vi "Chamber controller RT SAVE.vi"() -> ()   [LabVIEW 2014]
uses:
  <vilib>/Instr/_visa.llb/VISA Configure Serial Port (Instr).vi
  Environmental Chamber LabVIEW and Instruments/Drivers and Software/Keithley 2100 Series/Public/Configure/Configure 2 Wire Resistance.vi
  <vilib>/Utility/file.llb/Write To Spreadsheet File (string).vi
  <vilib>/Utility/file.llb/Read From Spreadsheet File (string).vi
  Environmental Chamber LabVIEW and Instruments/Drivers and Software/keithley_6430/Keithley 6430/Public/Data/Read (Single Point).vi
  Environmental Chamber LabVIEW and Instruments/Drivers and Software/LabVIEW 8.2 Drivers/keithley_24xx/Keithley 24XX/Public/Data/Read (Single Point).vi
  Environmental Chamber LabVIEW and Instruments/Drivers and Software/keithley_24xx/Keithley 24XX/Keithley 24XX.lvlib
  Environmental Chamber LabVIEW and Instruments/Drivers and Software/keithley_6430/Keithley 6430/Keithley 6430.lvlib
  Environmental Chamber LabVIEW and Instruments/Drivers and Software/Keithley 2100 Series/Keithley 2100 Series.lvlib
panel:
  out "saving data?":bool
  out "ArduinoQCM\ncluster":T1 caption="Arduino QCM" {"Freq 5" format="%#_10g"; "Freq 4" format="%#_10g"; "Freq 3" format="%#_10g"; "Freq 2" format="%#_10g"; "Freq 1" format="%#_10g"}
  in  "Data logging settings":T2={"Save during sequence only"=TRUE, "Save now"=FALSE, "sec between data points"=0.0, "Current data file path"=path "", "Save sample names"={"QCM1"="aQCM2", "QCM2"="aQCM2", "QCM3"="aQCM3", "QCM4"="aQCM4", "QCM5"="aQCM5", "QCM6"="aQCM6", "SRS"="sample_SRS", "K-2420"="Keithley2420", "K-6430"="Keithley6430", "K-2100"="Keithley2100"}, "Experiment Notes"=""} {"sec between data points" min=0.0 max=30.0 format="%#_13g"}
  in  "Sequence cluster":T3={"Save sequence"=FALSE, "Clear sequence"=FALSE, "Import sequence file"=FALSE, "Tare elapsed time"=TRUE, "Run Sequence"=FALSE, "Stop program when sequence ends"=TRUE, "User-defined\nsequence"=[], "Sequence end time"="", "Sequence\npreview"=[], "Current\nstep"=0, "Jump to next step"=FALSE} caption="Sequence settings"
  in  "Pressure parameters cluster":T4={"valve % open"=100.0, "Desired pressure"=0.0, "Vapor sccm"=0.0, "Gas sccm"=0.0, "Valve mode"=enum."% Open", "Pressure Mode"=enum."Abs. pressure", "analyte partial pressure"=23.8, "Turbo pump\nauto on"=TRUE, "Valve position (%)"=0.0, "read pressure"=0.0, "read vapor flow"=0.0, "read gas flow"=0.0, "pressure chart"={"pressure"=0.0}} caption="Pressure settings" {"read gas flow" format="%#_3g"; "read vapor flow" format="%#_3g"; "read pressure" format="%#_7f"; "Valve position (%)" format="%#_3g"; "analyte partial pressure" min=0.0 max=100.0 step=5.0; "Gas sccm" min=0 max=200 step=5; "Vapor sccm" min=0 max=200 step=5; "Desired pressure" min=0.0 max=760.0 step=5.0; "valve % open" min=0.0 max=100.0 step=5.0 format="%#_2f"}
  out "J-KEM temp chart":dbl(graph)
  out "Elapsed time (min)":dbl
  out "State date/time":string caption="Start time"
  out "K-2100 (Ohm)":cluster{"Measurement":dbl}(graph) caption="K-2100 Ohm"
  out "K-6430":cluster{"Measurement":dbl}(graph)
  out "K-2420":cluster{"Resistance":sgl}(graph)
  in  "Gate time (sec)":enum16{"0.1", "1.0 ", "10"}(ring)=enum."1.0 "
  out "MHz":dbl format="%.9f"
  out "QCM plot":T5(graph)
  in  "Stop":bool
  in  "Clear all charts":bool
  out "O2 sensor output":dbl[](array[numeric]) caption="atm\nTorr"
  in  "rapidox O2 Sensor":bool
  in  "setnag O2 Pump":bool
  in  "Baud Rate 2":i32(ring)=2 items=["2400", "4800", "9600", "19200", "38400", "57600", "115200"]
  in  "Com Port":i32(ring) items=["Com 1", "Com 2", "Com 3", "Com 4", "Com 5", "Com 6", "COM 7", "COM 8", "COM 9", "COM 10", "COM 11", "COM 12", "com 13", "COM 14"]
  in  "Com Port 2":i32(ring) items=["Com 1", "Com 2", "Com 3", "Com 4", "Com 5", "Com 6", "COM 7", "COM 8", "COM 9", "COM 10", "COM 11", "COM 12", "com 13", "COM 14"]
  out "Waveform Chart":cluster{dbl}(graph)
  out "O2 Concentration (PPM)":dbl
  out "Waveform Chart 6":cluster{dbl}(graph)
  # "Currently Unused"
  # "100%"
  # "SRS"
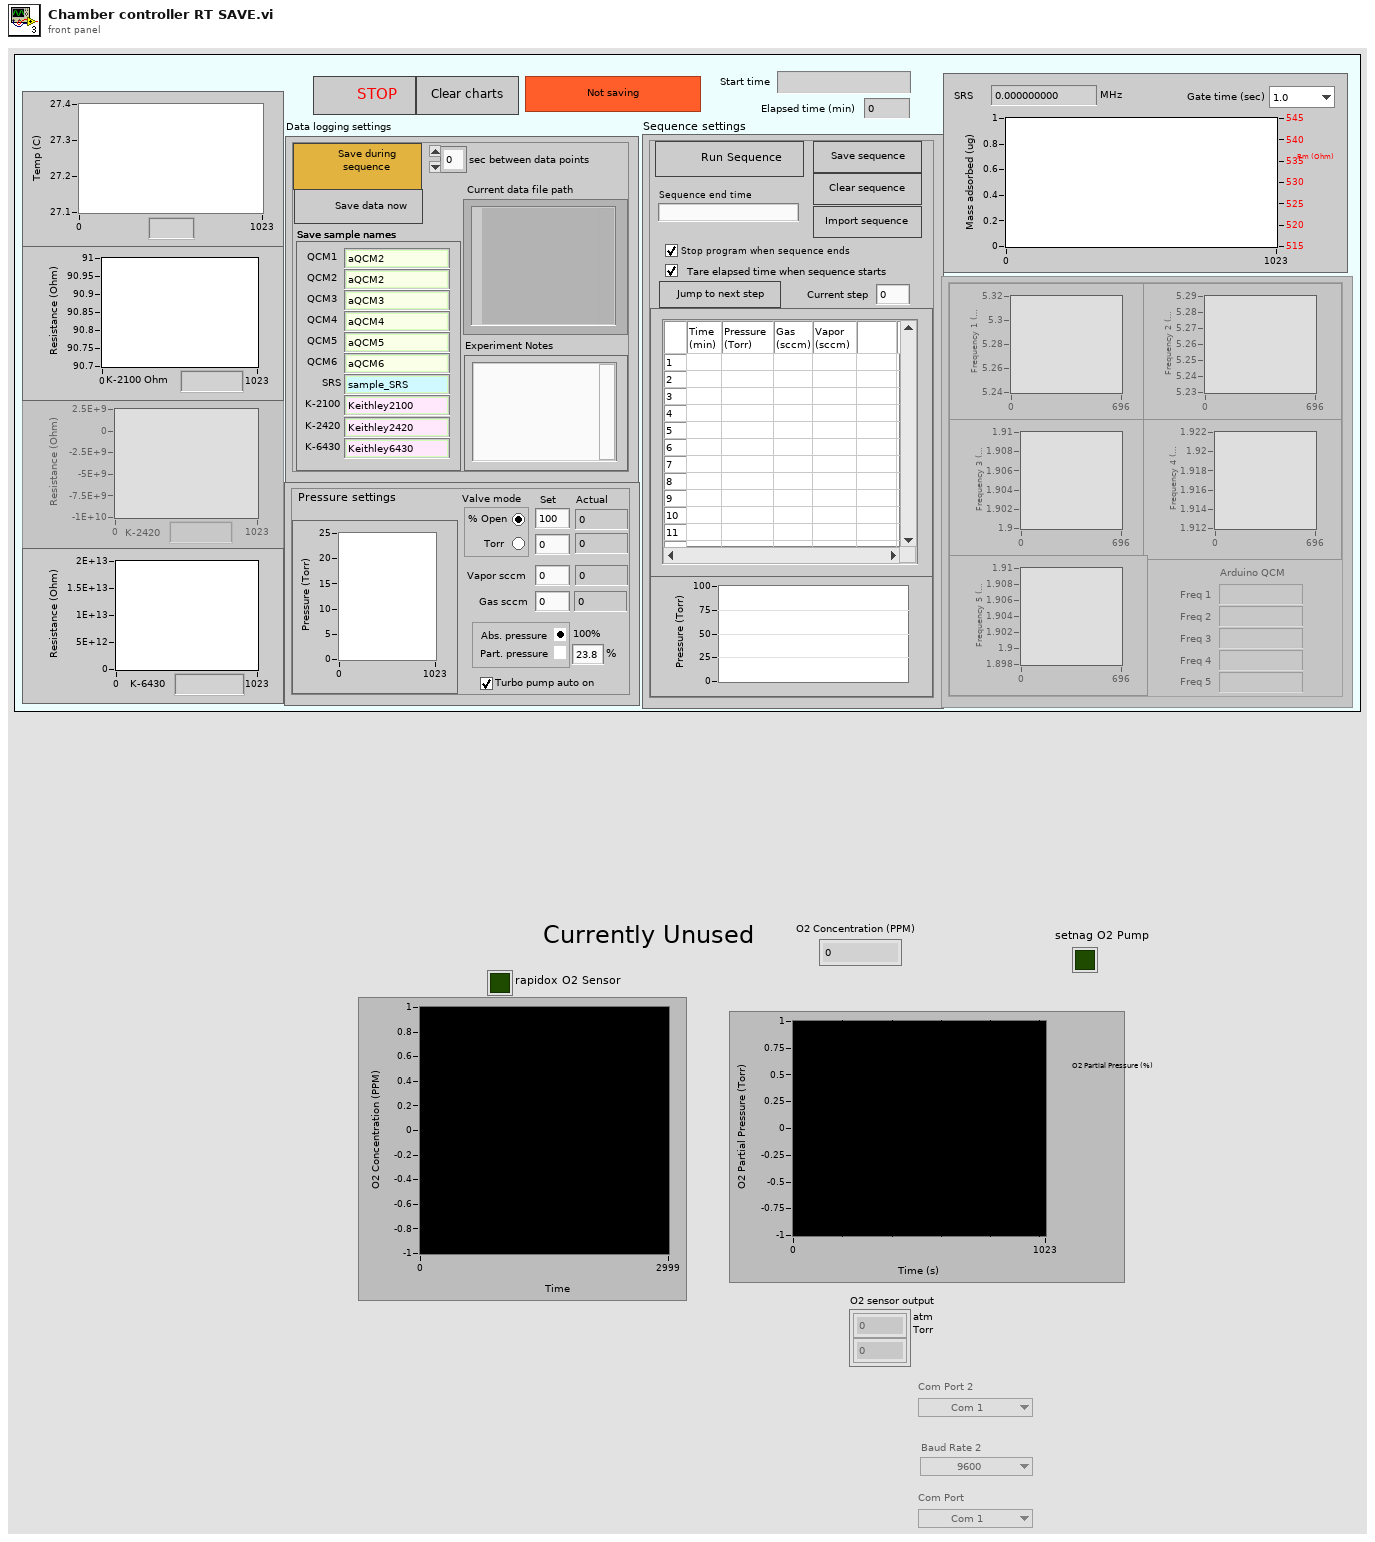
[diagram p1: front panel]
types:
  T1 = cluster{"arduino qcm 1":dbl, "Freq 1":dbl, "arduino qcm 2":dbl, "Freq 2":dbl, "arduino qcm 3":dbl, "Freq 3":dbl, "arduino qcm 4":dbl, "Freq 4":dbl, "arduino qcm 5":dbl, "Freq 5":dbl}
  T2 = cluster{"Save during sequence only":bool, "Save now":bool, "sec between data points":dbl, "Current data file path":path, "Save sample names":cluster{"QCM1":string, "QCM2":string, "QCM3":string, "QCM4":string, "QCM5":string, "QCM6":string, "SRS":string, "K-2420":string, "K-6430":string, "K-2100":string}, "Experiment Notes":string}
  T3 = cluster{"Save sequence":bool, "Clear sequence":bool, "Import sequence file":bool, "Tare elapsed time":bool, "Run Sequence":bool, "Stop program when sequence ends":bool, "User-defined\nsequence":string[][], "Sequence end time":string, "Sequence\npreview":cluster{dbl[], dbl[]}[], "Current\nstep":i32, "Jump to next step":bool}
  T4 = cluster{"valve % open":dbl, "Desired pressure":dbl, "Vapor sccm":sgl, "Gas sccm":sgl, "Valve mode":enum32{"% Open", "Torr "}, "Pressure Mode":enum32{"Abs. pressure", " Part. pressure"}, "analyte partial pressure":dbl, "Turbo pump\nauto on":bool, "Valve position (%)":dbl, "read pressure":dbl, "read vapor flow":dbl, "read gas flow":dbl, "pressure chart":cluster{"pressure":dbl}}
  T5 = cluster{"Numeric Control":dbl, "Resistance out":dbl}
  T6 = cluster{"Keithley 6430":bool, "J-KEM":bool, "Keithley 2420":bool, "Keithley 2100":bool, "SRS QCM":bool, "Pressure control":bool, "Arduino":bool}
  T7 = enum8{"Enabled", "Disabled", "Disabled and Grayed Out"}
  T8 = cluster{"Arduino 1":refnum<visa-resource-name>, "Arduino 2":refnum<visa-resource-name>, "Arduino 3":refnum<visa-resource-name>, "Arduino 4":refnum<visa-resource-name>, "Arduino 5":refnum<visa-resource-name>}
  T9 = enum16{"open", "open or create", "create or replace", "create", "open (read only)"}
  T10 = enum16{"no parity", "odd parity", "even parity", "mark parity", "space parity"}
  T11 = cluster{"f":dbl, "f":dbl, "f":dbl, "f":dbl, "f":dbl}
  T12 = cluster{"String":string, "String":string, "String":string}
  T13 = cluster{"task out":refnum<k21>, "error out":errorcluster, "task out":refnum<k21>, "error out":errorcluster, "task out":refnum<k21>, "error out":errorcluster, "VISA resource name":refnum<visa-resource-name>, "error out":errorcluster}
  T14 = cluster{"task out":refnum<k21>, "error out":errorcluster, "task out":refnum<k21>, "error out":errorcluster, "task out":refnum<k21>, "error out":errorcluster, "VISA resource name out":refnum<visa-resource-name>, "error out":errorcluster}
  T15 = cluster{bool, "VISA resource name":refnum<visa-resource-name>, "error out":errorcluster}
  T16 = cluster{bool, "VISA resource name out":refnum<visa-resource-name>, "error out":errorcluster}
  T17 = cluster{"VISA resource name out":refnum<visa-resource-name>, "error out":errorcluster, "VISA resource name out":refnum<visa-resource-name>, "error out":errorcluster, "VISA resource name out":refnum<visa-resource-name>, "error out":errorcluster, "VISA resource name out":refnum<visa-resource-name>, "error out":errorcluster, "VISA resource name out":refnum<visa-resource-name>, "error out":errorcluster}
  T18 = cluster{bool, cluster{"task out":refnum<k21>, "error out":errorcluster, "task out":refnum<k21>, "error out":errorcluster, "task out":refnum<k21>, "error out":errorcluster, "VISA resource name out":refnum<visa-resource-name>, "error out":errorcluster}}
  T19 = cluster{"Boolean":bool, "VISA resource name out":refnum<visa-resource-name>, "error out":errorcluster}
  T20 = cluster{bool, "VISA out":refnum<visa-resource-name>, "error out":errorcluster}
  T21 = cluster{"Boolean":bool, "VISA out":refnum<visa-resource-name>, "error out":errorcluster}
  T22 = cluster{"Numeric Control":dbl, "Cluster":cluster{"Numeric Control":dbl}, "String":string, "error out":errorcluster}
  T23 = cluster{bool, "Com Port":i32, "Numeric Control out":dbl}
  T24 = cluster{"VISA Refnum out":refnum<visa-resource-name>, "error out":errorcluster, "VISA Refnum out":refnum<visa-resource-name>, "error out":errorcluster, "VISA Refnum out":refnum<visa-resource-name>, "error out":errorcluster, "VISA Refnum out":refnum<visa-resource-name>, "error out":errorcluster, "VISA Refnum out":refnum<visa-resource-name>, "error out":errorcluster}
  T25 = cluster{"f":string, "f":string, "f":string, "f":string, "f":string}
  T26 = cluster{"String data out":string, string, string, string}
  T27 = cluster{"valve % open":dbl, "Desired pressure":dbl, "Vapor sccm":sgl, "Gas sccm":sgl, "Valve mode":enum32{"% Open", "Torr "}, "Pressure Mode":enum32{"Abs. pressure", " Part. pressure"}, "analyte partial pressure":dbl, "Turbo pump\nauto on":bool}
  T28 = cluster{"User-defined\nsequence":string[][], "Present (s)":dbl, "current  step # in":i32, "sequence end time in":timestamp}
  T29 = cluster{"current  step # in":i32, "sequence end time in":timestamp, "Boolean":bool}
  T30 = cluster{"press/RH/gas/vapor":cluster{"pressure":string, "RH":string, "gas flow":string, "vapor flow":string}, "Cluster":cluster{"Valve position (%)":dbl, "read pressure":dbl, "read vapor flow":dbl, "read gas flow":dbl}}
  T31 = cluster{"Boolean":bool, "DAQ IDs in":cluster{"task out":refnum<k21>, "error out":errorcluster, "task out":refnum<k21>, "error out":errorcluster, "task out":refnum<k21>, "error out":errorcluster, "VISA Refnum out":refnum<visa-resource-name>, "error out":errorcluster}}
  T32 = cluster{"f":dbl, "f":dbl, "f":dbl, "f":dbl, "f":dbl}[]
  T33 = cluster{"pressure":string, "RH":string, "gas flow":string, "vapor flow":string}
  T34 = cluster{"Valve position (%)":dbl, "read pressure":dbl, "read vapor flow":dbl, "read gas flow":dbl}
  T35 = cluster{"f":dbl, "f":dbl, "f":dbl, "f":dbl, "f":dbl, "f":dbl, "f":dbl, "f":dbl, "f":dbl, "f":dbl}
  T36 = cluster{"QCM1":string, "QCM2":string, "QCM3":string, "QCM4":string, "QCM5":string, "QCM6":string, "SRS":string, "K-2420":string, "K-6430":string, "K-2100":string}
  T37 = cluster{"task out":refnum<k21>, "error out":errorcluster, "task out":refnum<k21>, "error out":errorcluster, "task out":refnum<k21>, "error out":errorcluster, "VISA Refnum out":refnum<visa-resource-name>, "error out":errorcluster}
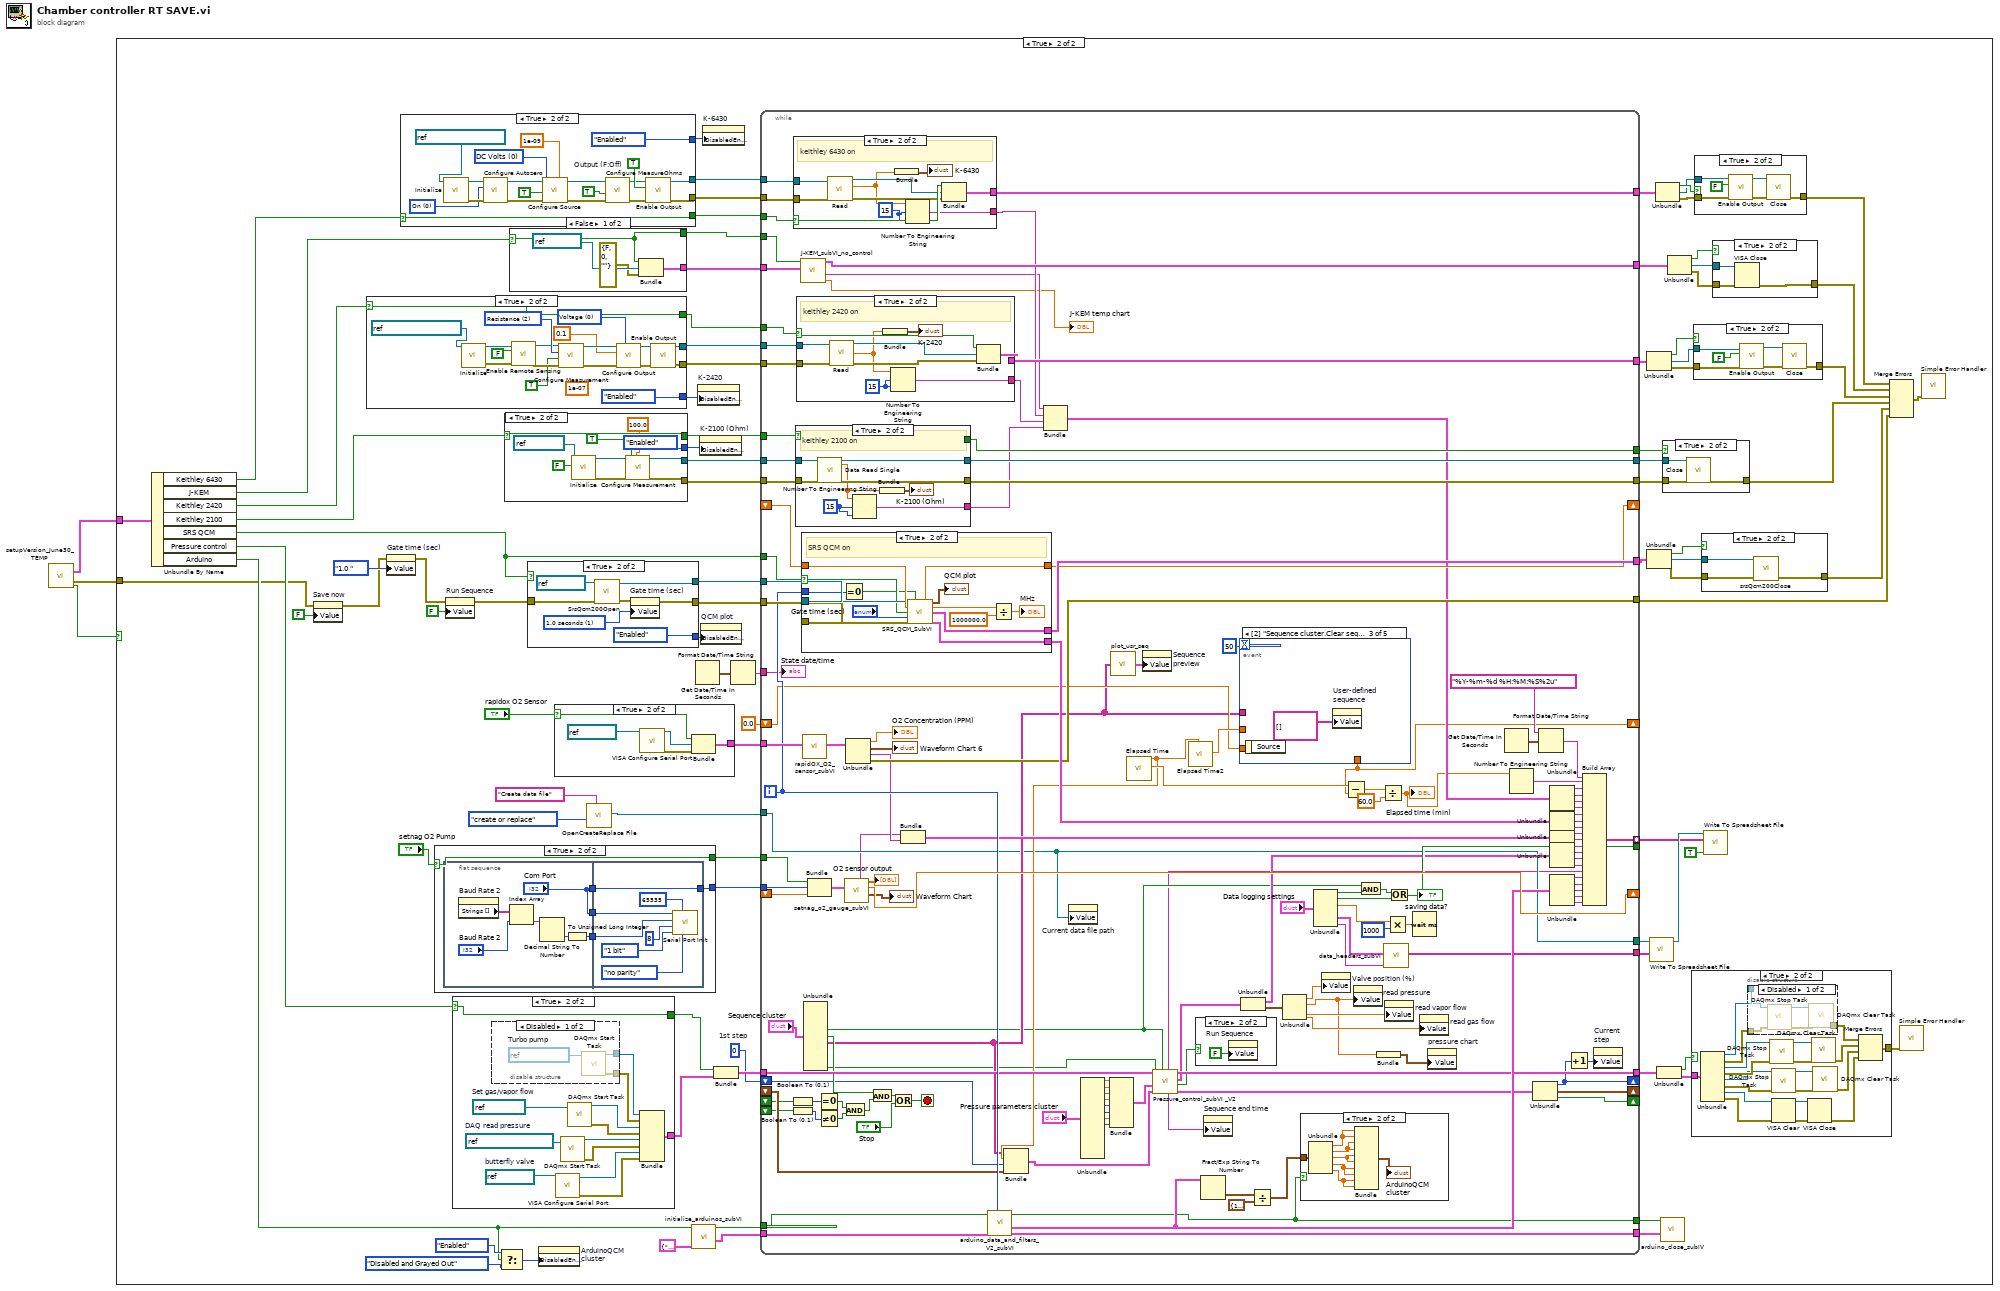
[diagram p0: block diagram]
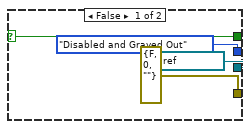
[diagram p4: hidden frame]
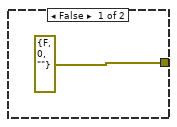
[diagram p5: hidden frame]
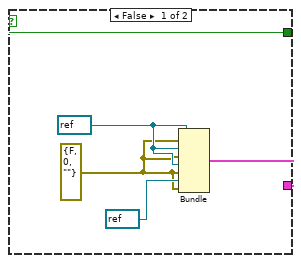
[diagram p7: hidden frame]
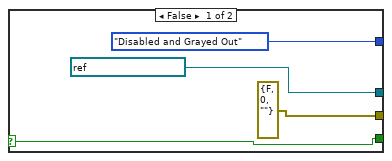
[diagram p10: hidden frame]
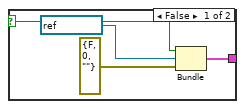
[diagram p11: hidden frame]
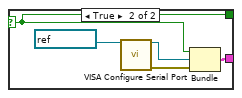
[diagram p13: hidden frame]
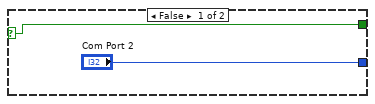
[diagram p14: hidden frame]
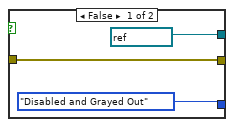
[diagram p16: hidden frame]
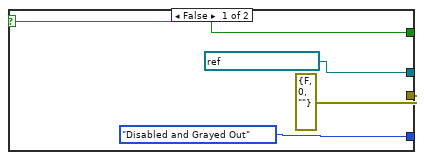
[diagram p18: hidden frame]
diagram:
  n1 = call "setupVersion_June30_TEMP.vi"() -> ("Instruments on/off"=w1:T6, "error IO"=w2:errorcluster, "OK"=w3:bool)  [unwired: 13 in]
  n2 = case shown="True" w3 {
    tunnel: w2 -> [_ w6]
    tunnel: w1 -> [_ w14]
    frame False {
    }
    frame True {
      w26 = 0  # 1st step
      n3 = Unbundle By Name(w14) -> ("Keithley 6430"=w13:bool, "J-KEM"=w12:bool, "Keithley 2420"=w11:bool, "Keithley 2100"=w10:bool, "SRS QCM"=w9:bool, "Pressure control"=w8:bool, "Arduino"=w7:bool)
      n4 = property on="Save now" class="Bool (strict)"(error in=w6, "Value"=FALSE) -> (error out=w5:errorcluster)  [unwired: 1 in, 1 out]
      n5 = case shown="True" w11 {
        selector: w11 -> [w252 w256]
        tunnel: [refnum<visa-resource-name> "GPIB1::24::INSTR" ("VISA resource name") w265] -> w91
        tunnel: [errorcluster {"status"=FALSE, "code"=0, "source"=""} ("error out") w260] -> w90
        tunnel: [T7."Disabled and Grayed Out" ("Disabled") T7."Enabled" ("Disabled")] -> w54
        tunnel: [w252 w256] -> w47
        frame False {
        }
        frame True {
          (unwired) 1e-07 ("Manual Range (1.0)")
          w267 = u16 0 items=["Voltage", "Current"] ("Source Mode  (0: Voltage)")
          w272 = u16 2 items=["Volts", "Current", "Resistance"] ("Function (0: Volts)")
          n6 = call "Initialize.vi"("VISA resource name"=refnum<visa-resource-name> "GPIB1::24::INSTR") -> ("error out"=w261:errorcluster, "VISA resource name out"=w264:refnum<visa-resource-name>)  [unwired: 9 in]
          n7 = call "Enable Remote Sensing.vi"("error in (no error)"=w261, "Enable Remote Sensing (T: Enable)"=FALSE ("4-wire?"), "VISA resource name"=w264) -> ("error out"=w262:errorcluster, "VISA resource name out"=w263:refnum<visa-resource-name>)  [unwired: 7 in]
          n8 = call "Configure Measurement.vi"("error in (no error)"=w262, "Enable Auto Range (T:Enable)"=TRUE, "Function (0: Volts)"=w272, "VISA resource name"=w263) -> ("error out"=w271:errorcluster, "VISA resource name out"=w270:refnum<visa-resource-name>)  [unwired: 6 in]
          n9 = call "Configure Output.vi"("Source Mode  (0: Voltage)"=w267, "error in (no error)"=w271, "Output Level (0)"=0.1 ("Applied Voltage (V)"), "VISA resource name"=w270) -> ("error out"=w269:errorcluster, "VISA resource name out"=w268:refnum<visa-resource-name>)  [unwired: 6 in]
          n10 = call "Enable Output.vi"("error in (no error)"=w269, "VISA resource name"=w268) -> ("error out"=w260:errorcluster, "VISA resource name out"=w265:refnum<visa-resource-name>)  [unwired: 8 in]
        }
      }
      n11 = property on="Gate time (sec)" class="Enum (strict)"(error in=w5, "Value"=enum16{"0.1", "1.0 ", "10"}."1.0 " ("Gate time (sec)")) -> (error out=w15:errorcluster)  [unwired: 1 in, 1 out]
      n12 = case shown="True" w13 {
        selector: w13 -> [w166 w170]
        tunnel: [refnum<visa-resource-name> "GPIB0::29::INSTR" ("VISA resource name") w183] -> w60
        tunnel: [errorcluster {"status"=FALSE, "code"=0, "source"=""} ("error out") w184] -> w59
        tunnel: [T7."Disabled and Grayed Out" ("Disabled") T7."Enabled" ("Disabled")] -> w53
        tunnel: [w166 w170] -> w46
        frame False {
        }
        frame True {
          w172 = u16 0 items=["DC Volts", "DC Current"] ("Source Function (0: DC Volts)")
          w179 = u16 0 items=["On", "Off", "Once"] ("Autozero  (0: On)")
          w187 = TRUE  # Output (F:Off)
          n13 = call "Initialize.vi"("VISA resource name"=refnum<visa-resource-name> "GPIB0::30::INSTR") -> ("error out"=w180:errorcluster, "VISA resource name out"=w181:refnum<visa-resource-name>)  [unwired: 4 in, 5 out]
          n14 = call "Configure Autozero.vi"("error in (no error)"=w180, "Autozero  (0: On)"=w179, "VISA resource name"=w181) -> ("error out"=w175:errorcluster, "VISA resource name out"=w177:refnum<visa-resource-name>)  [unwired: 7 in]
          n15 = call "Configure Source.vi"("I-Source Level [A]"=1e-09, "error in (no error)"=w175, "Auto Range (T:Enable)"=TRUE, "Source Function (0: DC Volts)"=w172, "VISA resource name"=w177) -> ("error out"=w174:errorcluster, "VISA resource name out"=w176:refnum<visa-resource-name>)  [unwired: 5 in]
          n16 = call "Configure MeasureOhms.vi"("error in (no error)"=w174, "Auto Range (T:Enable)"=TRUE, "VISA resource name"=w176) -> ("error out"=w188:errorcluster, "VISA resource name out"=w186:refnum<visa-resource-name>)  [unwired: 3 in, 4 out]
          n17 = call "Enable Output.vi"("error in (no error)"=w188, "Enable Output (F:Off)"=w187, "VISA resource name"=w186) -> ("error out"=w184:errorcluster, "VISA resource name out"=w183:refnum<visa-resource-name>)  [unwired: 7 out]
        }
      }
      n18 = case shown="True" "setnag O2 Pump" {
        selector: "setnag O2 Pump" -> [w211 w213]
        tunnel: ["Com Port 2" w214] -> w87
        tunnel: [w211 w213] -> w35
        frame False {
        }
        frame True {
          n19 = flat-sequence {
            tunnel: ["Com Port"] -> w217
            tunnel: [w219] -> w216
            tunnel: ["Com Port"] -> w215
            tunnel: w217 -> [w225]
            tunnel: w216 -> [w224]
            tunnel: w215 -> [w226]
            tunnel: [w226] -> w214
            frame #0 {
              n20 = property on="Baud Rate 2" class="Ring (strict)"() -> ("Strings []"=w221:string[])  [unwired: 2 in, 2 out]
              n21 = Index Array(array=w221, index="Baud Rate 2") -> (element=w222:string)
              n22 = Decimal String To Number(string=w222) -> (number=w220:i32)  [unwired: 2 in, 1 out]
              n23 = To Unsigned Long Integer(number=w220) -> (unsigned 32bit integer=w219:u32)
            }
            frame #1 {
              n24 = call <vilib>:"Serial Port Init.vi"("parity"=T10."no parity", "buffer size"=u16 65535, "stop bits"=enum16{"1 bit", "1.5 bits", "2 bits"}."1 bit", "data bits"=u16 8, "baud rate"=w224, "port number"=w225) -> ()  [unwired: 1 in, 1 out]
            }
          }
        }
      }
      n25 = property on="Run Sequence" class="Bool (strict)"(error in=w15, "Value"=FALSE) -> (error out=w21:errorcluster)  [unwired: 1 in, 1 out]
      n26 = case shown="True" w8 {
        selector: w8 -> [w138 w143]
        tunnel: [w139 w145] -> w28
        tunnel: [w138 w143] -> w29
        frame False {
          w141 = refnum<k21> refnum ("task out")
          w140 = errorcluster {"status"=FALSE, "code"=0, "source"=""} ("error out")
          n27 = Bundle("task out"=w141, "error out"=w140, "task out"=w141, "error out"=w140, "task out"=w141, "error out"=w140, "VISA resource name"=refnum<visa-resource-name> refnum, "error out"=w140) -> (w139:T13)  [unwired: 1 in]
        }
        frame True {
          w153 = refnum<visa-resource-name> "COM5"  # butterfly valve
          w154 = refnum<k21> "Setflow"  # Set gas/vapor flow
          w155 = refnum<k21> "AllDaqReadings"  # DAQ read pressure
          n28 = disable-structure shown="Disabled" {
            disable-tunnel: [w157 _] -> w152
            disable-tunnel: [w156 _] -> w151
            frame Disabled {
              w158 = refnum<k21> "TurboON"  # Turbo pump
              n29 = call <vilib>:"DAQmx Start Task.vi"("task/channels in"=w158) -> ("task out"=w157:refnum<k21>, "error out"=w156:errorcluster)  [unwired: 13 in]
            }
            frame Enabled {
            }
          }
          n30 = call-poly "VISA Configure Serial Port"("VISA resource name"=w153) -> ("VISA resource name out"=w146:refnum<visa-resource-name>, "error out"=w144:errorcluster)  [unwired: 13 in]
          n31 = call <vilib>:"DAQmx Start Task.vi"("task/channels in"=w155) -> ("task out"=w148:refnum<k21>, "error out"=w147:errorcluster)  [unwired: 13 in]
          n32 = call <vilib>:"DAQmx Start Task.vi"("task/channels in"=w154) -> ("task out"=w150:refnum<k21>, "error out"=w149:errorcluster)  [unwired: 13 in]
          n33 = Bundle("task out"=w152, "error out"=w151, "task out"=w150, "error out"=w149, "task out"=w148, "error out"=w147, "VISA resource name out"=w146, "error out"=w144) -> (w145:T14)  [unwired: 1 in]
        }
      }
      n34 = Select(t=T7."Enabled" ("Disabled"), s=w7, f=T7."Disabled and Grayed Out" ("Disabled")) -> (s? t:f=w20:T7)
      n35 = case shown="True" w10 {
        selector: w10 -> [w99 w105]
        tunnel: [refnum<visa-resource-name> "K-2100" ("VISA resource name out") w108] -> w44
        tunnel: [errorcluster {"status"=FALSE, "code"=0, "source"=""} ("error out") w107] -> w43
        tunnel: [w99 w105] -> w42
        tunnel: [T7."Disabled and Grayed Out" ("Disabled") T7."Enabled" ("Disabled")] -> w37
        frame False {
        }
        frame True {
          n36 = call "Initialize.vi"("VISA resource name"=refnum<visa-resource-name> "K-2100", "Reset? (T: Reset)"=FALSE) -> ("VISA resource name out"=w109:refnum<visa-resource-name>, "error out"=w106:errorcluster)  [unwired: 16 in]
          n37 = call-poly "Configure Measurement.vi"("VISA resource name"=w109, "error in (no error)"=w106, "Auto Range? (T: Auto)"=TRUE, "Custom Range (100 Ohm)"=100.0 ("Temp (C) 2")) -> ("VISA resource name out"=w108:refnum<visa-resource-name>, "error out"=w107:errorcluster)  [unwired: 14 in]
        }
      }
      n38 = case shown="False" w12 {
        selector: w12 -> [w202 w207]
        tunnel: [w203 w208] -> w76
        tunnel: [w202 w207] -> w70
        frame False {
          n39 = Bundle(w202, "VISA resource name"=refnum<visa-resource-name> "COM3", "error out"=errorcluster {"status"=FALSE, "code"=0, "source"=""}) -> (w203:T15)  [unwired: 1 in]
        }
        frame True {
          n40 = call-poly "VISA Configure Serial Port"("VISA resource name"=refnum<visa-resource-name> "COM3") -> ("VISA resource name out"=w209:refnum<visa-resource-name>, "error out"=w206:errorcluster)  [unwired: 13 in]
          n41 = Bundle(w207, "VISA resource name out"=w209, "error out"=w206) -> (w208:T16)  [unwired: 1 in]
        }
      }
      n42 = case shown="True" w9 {
        tunnel: [refnum<visa-resource-name> "COM6" ("VISA in") w241] -> w89
        tunnel: [w236 w238] -> w88
        tunnel: w21 -> [w236 w243]
        tunnel: [T7."Disabled and Grayed Out" ("Disabled") T7."Enabled" ("Disabled")] -> w55
        frame False {
        }
        frame True {
          w240 = u16 1 items=["0.1 seconds", "1.0 seconds", "10.0 seconds"] ("Gate time")
          n43 = call "SrsQcm200Open.vi"("error in"=w243, "VISA in"=refnum<visa-resource-name> "COM6") -> ("error out"=w239:errorcluster, "VISA out"=w241:refnum<visa-resource-name>)  [unwired: 3 in]
          n44 = property on="Gate time (sec)" class="Enum (strict)"(error in=w239, "Value"=w240) -> (error out=w238:errorcluster)  [unwired: 1 in, 1 out]
        }
      }
      n45 = property on="ArduinoQCM\ncluster" class="Clust (strict)"("DisabledEnum"=w20) -> ()  [unwired: 2 in, 2 out]
      n46 = case shown="True" "rapidox O2 Sensor" {
        selector: "rapidox O2 Sensor" -> [w189 w194]
        tunnel: [w190 w195] -> w66
        frame False {
          n47 = Bundle(w189, "VISA resource name"=refnum<visa-resource-name> "COM7", "error out"=errorcluster {"status"=FALSE, "code"=0, "source"=""}) -> (w190:T15)  [unwired: 1 in]
        }
        frame True {
          n48 = call-poly "VISA Configure Serial Port"("VISA resource name"=refnum<visa-resource-name> "COM7") -> ("VISA resource name out"=w196:refnum<visa-resource-name>, "error out"=w193:errorcluster)  [unwired: 13 in]
          n49 = Bundle(w194, "VISA resource name out"=w196, "error out"=w193) -> (w195:T16)  [unwired: 1 in]
        }
      }
      n50 = call "OpenCreateReplace File.vi"("prompt"="Create data file", "function (open:0)"=T9."create or replace") -> ("new file path"=w45:path)  [unwired: 6 in, 3 out]
      n51 = call "initialize_arduinos_subVI.vi"("arduino 1-6 addresses"=T8 {"Arduino 1"="COM21", "Arduino 2"="COM22", "Arduino 3"="COM23", "Arduino 4"="COM24", "Arduino 5"="COM26"}, "arduinos on?"=w7) -> ("arduino addresses/errors"=w30:T17, "arduinos on/off"=w51:bool)  [unwired: 8 in]
      n52 = Get Date/Time In Seconds() -> (seconds since 1Jan1904=w93:timestamp)
      n53 = property on="K-2420" class="WFChart (strict)"("DisabledEnum"=w54) -> ()  [unwired: 2 in, 2 out]
      n54 = property on="K-2100 (Ohm)" class="WFChart (strict)"("DisabledEnum"=w37) -> ()  [unwired: 2 in, 2 out]
      n55 = property on="QCM plot" class="WFChart (strict)"("DisabledEnum"=w55) -> ()  [unwired: 2 in, 2 out]
      n56 = property on="K-6430" class="WFChart (strict)"("DisabledEnum"=w53) -> ()  [unwired: 2 in, 2 out]
      n57 = Bundle(w29, w28) -> (w27:T18)  [unwired: 1 in]
      n58 = Format Date/Time String(seconds (now)=w93) -> (date/time string=w34:string)  [unwired: 2 in]
      n59 = while {
        shift-right: [w418] -> _
        shift-left: _ -> [w340]
        tunnel: [w402] -> w52 mode=indexing if=w366
        tunnel: w47 -> [w407]
        tunnel: w91 -> [w417]
        tunnel: w90 -> [w416]
        tunnel: w89 -> [w415]
        tunnel: w88 -> [w414]
        tunnel: w9 -> [w413]
        tunnel: w35 -> [w342]
        tunnel: w87 -> [w343]
        tunnel: [w412] -> w84
        tunnel: [w411] -> w80
        tunnel: w76 -> [w410]
        tunnel: [w409] -> w75
        tunnel: w70 -> [w408]
        tunnel: w66 -> [w354]
        tunnel: [w350] -> w32
        tunnel: [w282] -> w65
        tunnel: w45 -> [w282]
        shift-right: [w400] -> _
        shift-left: _ -> [w401]
        tunnel: w60 -> [w406]
        tunnel: w59 -> [w405]
        tunnel: [w404] -> w58
        tunnel: [w366] -> _
        tunnel: w51 -> [w349]
        tunnel: w30 -> [w393]
        tunnel: [w348] -> w49
        tunnel: [w392] -> w50
        tunnel: [w385] -> w48
        tunnel: w46 -> [w378]
        tunnel: w44 -> [w365]
        tunnel: w43 -> [w364]
        tunnel: w42 -> [w363]
        tunnel: [w362] -> w41
        tunnel: [w361] -> w40
        tunnel: [w360] -> w39
        shift-right: [w334] -> _
        shift-left: 0.0 ("Elapsed Time (s)") -> [w335]
        tunnel: w34 -> [w325]
        tunnel: w27 -> [w307]
        shift-right: [w277] -> _
        shift-left: w26 -> [w296]
        shift-right: [w302] -> _
        shift-left: _ -> [w300]
        shift-right: [w301] -> _
        shift-left: _ -> [w299]
        shift-left: _ -> [w298]
        tunnel: [w294] -> w25
        i -> [w344]
        stop <- w368 stop-if-true
        n60 = Boolean To (0,1)(Boolean=w299) -> (0, 1=w376:i16)
        n61 = Boolean To (0,1)(Boolean=w298) -> (0, 1=w375:i16)
        n62 = case "Keithley 6430" shown="True" w378 {
          selector: w378 -> [w452 w463]
          tunnel: w406 -> [w451 w460]
          tunnel: w405 -> [w450 w459]
          tunnel: ["" w462] -> w347
          tunnel: [w449 w461] -> w404
          frame False {
            # "keithley 6430 off"
            n63 = Bundle(w452, "VISA resource name out"=w451, "error out"=w450) -> (w449:T16)  [unwired: 1 in]
          }
          frame True {
            w454 = i16 15 ("width (-)")
            # "keithley 6430 on"
            n64 = call-poly "Read.vi"("error in (no error)"=w459, "VISA resource name"=w460) -> ("error out"=w458:errorcluster, "Measurement"=w456:dbl, "VISA resource name out"=w457:refnum<visa-resource-name>)  [unwired: 1 in, 6 out]
            n65 = Bundle("Measurement"=w456) -> (→"K-6430":cluster{"Measurement":dbl})  [unwired: 1 in]
            n66 = Number To Engineering String(2:w454, 3:w454, 4:w456) -> (0:w462:string)  [unwired: 1 in]
            n67 = Bundle(w463, "VISA resource name out"=w457, "error out"=w458) -> (w461:T16)  [unwired: 1 in]
          }
        }
        n68 = case shown="True" w363 {
          selector: w363 -> [w428 w433]
          tunnel: [w429 w440] -> w361
          tunnel: [w430 w439] -> w360
          tunnel: w365 -> [w429 w438]
          tunnel: w364 -> [w430 w437]
          tunnel: ["" w435] -> w345
          tunnel: [w428 w433] -> w362
          frame False {
            # "keithley 2100 off"
          }
          frame True {
            w432 = i16 15 ("width (-)")
            # "keithley 2100 on"
            n69 = call "Data Read Single.vi"("VISA resource name"=w438, "error in (no error)"=w437) -> ("VISA resource name out"=w440:refnum<visa-resource-name>, "Measurement"=w436:dbl, "error out"=w439:errorcluster)  [unwired: 15 in]
            n70 = Number To Engineering String ("elapsed time (min)")(2:w432, 3:w432, 4:w436) -> (0:w435:string)  [unwired: 1 in]
            n71 = Bundle("Measurement"=w436) -> (→"K-2100 (Ohm)":cluster{"Measurement":dbl})  [unwired: 1 in]
          }
        }
        n72 = case "Keithley 2420" shown="True" w407 {
          selector: w407 -> [w467 w476]
          tunnel: w417 -> [w466 w471]
          tunnel: w416 -> [w465 w470]
          tunnel: [w464 w474] -> w412
          tunnel: ["" w473] -> w346
          frame False {
            # "keithley 2420 off"
            n73 = Bundle(w467, "VISA resource name out"=w466, "error out"=w465) -> (w464:T16)  [unwired: 1 in]
          }
          frame True {
            w469 = i16 15 ("width (-)")
            # "keithley 2420 on"
            n74 = call-poly "Read.vi"("VISA resource name"=w471, "error in (no error)"=w470) -> ("VISA resource name out"=w477:refnum<visa-resource-name>, "Resistance"=w472:sgl, "error out"=w475:errorcluster)  [unwired: 7 in, 4 out]
            n75 = Bundle("Resistance"=w472) -> (→"K-2420":cluster{"Resistance":sgl})  [unwired: 1 in]
            n76 = Number To Engineering String(2:w469, 3:w469, 4:w472) -> (0:w473:string)  [unwired: 1 in]
            n77 = Bundle(w476, "VISA resource name out"=w477, "error out"=w475) -> (w474:T16)  [unwired: 1 in]
          }
        }
        n78 = call "J-KEM_subVI_no_control.vi"("Address in"=w410, "J-KEM on?"=w408) -> ("Temp (C)"=→"J-KEM temp chart":dbl, "String data out"=w333:string, "Address out"=w409:T19)  [unwired: 6 in, 1 out]
        n79 = case "SRS QCM" shown="True" w413 {
          selector: w413 -> [w481 w492]
          tunnel: w415 -> [w484 w494]
          tunnel: w414 -> [w483 w495]
          tunnel: [w482 w498] -> w411
          tunnel: w401 -> [w479 w497]
          tunnel: [w479 w496] -> w400
          tunnel: [T12 {"String"="", "String"="", "String"=""} ("M,F,MR output cluster") w491] -> w390
          tunnel: w344 -> [_ w485]
          frame False {
            # "SRS QCM off"
            n80 = Bundle(w481, "VISA out"=w484, "error out"=w483) -> (w482:T20)  [unwired: 1 in]
          }
          frame True {
            # "SRS QCM on"
            n81 = Equal To 0?(x=w485) -> (x = 0?=w486:bool)
            n82 = call "SRS_QCM_SubVI.vi"("VISA Refnum in"=w494, "first iteration?"=w486, "Frequency out 3"=w497, "Boolean 2"=w492, "Gate time"="Gate time (sec)", "error in (no error)"=w495) -> ("Frequency out 2"=w496:dbl, "Cluster"=→"QCM plot":T5, "Frequency out"=w487:dbl, "Cluster 2"=w498:T21, "M,F,MR output cluster"=w491:T12)  [unwired: 2 in, 3 out]
            n83 = Divide(x=w487, y=1000000.0) -> (x/y=→"MHz":dbl)
          }
        }
        n84 = call "rapidOX_O2_sensor_subVI.vi"("rapid ox info in"=w354) -> ("rapidox info out"=w353:T22)  [unwired: 10 in]
        n85 = Unbundle("Sequence cluster") -> ("Run Sequence"=w288:bool, "Stop program when sequence ends"=w297:bool, "User-defined\nsequence"=w292:string[][], "Jump to next step"=w278:bool)  [unwired: 7 out]
        n86 = Bundle(w342, "Com Port"=w343, "Numeric Control out"=w340) -> (w341:T23)  [unwired: 1 in]
        n87 = Equal To 0?(x=w376) -> (x = 0?=w373:bool)
        n88 = Not Equal To 0?(x=w375) -> (x != 0?=w374:bool)
        n89 = And(x=w373, y=w374) -> (x .and. y?=w367:bool)
        n90 = call "setnag_o2_gauge_subVI.vi"("setnag info in"=w341) -> ("Cluster"=→"Waveform Chart":cluster{"Numeric Control":dbl}, "Numeric Control out"=w418:dbl, "Array"=→"O2 sensor output":dbl[], "String"=w279:string)  [unwired: 7 in]
        n91 = Unbundle(w353) -> ("Numeric Control"=→"O2 Concentration (PPM)":dbl, "Cluster"=→"Waveform Chart 6":cluster{"Numeric Control":dbl}, "String"=w324:string, "error out"=w350:errorcluster)
        n92 = And(x=w297, y=w367) -> (x .and. y?=w338:bool)
        n93 = Or(x=w338, y="Stop") -> (x .or. y?=w368:bool)
        n94 = Bundle("String"=w279, "String"=w324) -> (w323:cluster{"String":string, "String":string})  [unwired: 1 in]
        n95 = call "arduino_data_and_filters_V2_subVI.vi"("loop iteration number"=w344, "arduino 1-6 address and errors"=w393, "arduinos on?"=w349) -> ("arduino 1-6 addresses and errors out"=w392:T24, "arduino 1-6 data out"=w391:T25, "arduinos on? output"=w348:bool)  [unwired: 6 in]
        n96 = Bundle("String data out"=w333, w347, w346, w345) -> (w339:T26)  [unwired: 1 in]
        n97 = property on="Current data file path" class="Path"("Value"=w282) -> ()  [unwired: 2 in, 2 out]
        n98 = Unbundle("Pressure parameters cluster") -> ("valve % open"=w312:dbl, "Desired pressure"=w314:dbl, "Vapor sccm"=w315:sgl, "Gas sccm"=w316:sgl, "Valve mode"=w317:enum32{"% Open", "Torr "}, "Pressure Mode"=w318:enum32{"Abs. pressure", " Part. pressure"}, "analyte partial pressure"=w319:dbl, "Turbo pump\nauto on"=w320:bool)  [unwired: 5 out]
        n99 = Bundle("valve % open"=w312, "Desired pressure"=w314, "Vapor sccm"=w315, "Gas sccm"=w316, "Valve mode"=w317, "Pressure Mode"=w318, "analyte partial pressure"=w319, "Turbo pump\nauto on"=w320) -> (w311:T27)  [unwired: 1 in]
        n100 = call "plot_usr_seq.vi"("User-defined sequence"=w292) -> ("Sequence Preview"=w284:cluster{dbl[], dbl[]}[])
        n101 = call "Elapsed Time"() -> ("Present (s)"=w304:dbl, "Elapsed Time (s)"=w356:dbl)  [unwired: 12 in, 6 out]
        n102 = Bundle("User-defined\nsequence"=w292, "Present (s)"=w304, "current  step # in"=w296, "sequence end time in"=w300) -> (w305:T28)  [unwired: 1 in]
        n103 = property on="Sequence\npreview" class="XYGraph (strict)"("Value"=w284) -> ()  [unwired: 2 in, 2 out]
        n104 = call "Pressure_control_subVI _V2.vi"("Run Sequence"=w288, "user sequence, present (s) in, current step in, seq time in"=w305, "pressure parameters in"=w311, "Jump to next step"=w278, "pressure control on? / DAQ IDs/errors in"=w307) -> ("current step # out, shift register time out, seq button on?"=w303:T29, "sequence over? USE THIS TO REINITIALIZE RUN SEQUENCE BUTTON SO PROGRAM ENDS"=w293:bool, "save press/RH/gasflow/vaporflow - read valve position/pressure/vaporflow/gasflow"=w291:T30, "pressure control on out, DAQ IDs/errors out"=w294:T31, "sequence end date/time string"=w295:string, "pressure_setpoint"=w274:string)  [unwired: 1 in]
        n105 = call "Elapsed Time2"("Set Start Time (s)"=w304) -> ("Elapsed Time (s)"=w336:dbl)  [unwired: 11 in, 7 out]
        n106 = case shown="True" w293 {
          frame False {
          }
          frame True {
            n107 = property on="Run Sequence" class="Bool (strict)"("Value"=FALSE ("Run Sequence")) -> ()  [unwired: 2 in, 2 out]
          }
        }
        n108 = Fract/Exp String To Number(string=w391) -> (number=w384:T11)  [unwired: 3 in, 1 out]
        n109 = property on="Sequence end time" class="Str"("Value"=w295) -> ()  [unwired: 2 in, 2 out]
        n110 = event shown="[2] \"Sequence cluster.Clear sequence\": Value Change" {
          selector: _ -> [_ _ _ _ _]
          dyn-events: _ -> [_ _ _ _ _]
          timeout: 50 -> [_ _ _ _ _]
          tunnel: w292 -> [_ _ _ w447 _]
          tunnel: w336 -> [_ _ _ _ _]
          tunnel: w335 -> [w441 _ _ _ _]
          tunnel: [w441 _ _ _ _] -> w334
          event Timeout {
            n111 = event-data() -> ()  [unwired: 1 in, 1 out]
          }
          event "Clear all charts": Value Change {
            (unwired) T32 [] ("History Data")
            w444 = cluster{dbl}[] [] ("History Data")
            w445 = cluster{"Resistance":sgl}[] [] ("History Data")
            w443 = dbl[] [] ("History Data")
            n112 = event-data() -> ()  [unwired: 1 in, 1 out]
            n113 = property on="K-6430" class="WFChart (strict)"("History Data"=w445) -> ()  [unwired: 2 in, 2 out]
            n114 = property on="arduino qcm 3" class="WFChart (strict)"("History Data"=w443) -> ()  [unwired: 2 in, 2 out]
            n115 = property on="arduino qcm 1" class="WFChart (strict)"("History Data"=w443) -> ()  [unwired: 2 in, 2 out]
            n116 = property on="Waveform Chart" class="WFChart (strict)"("History Data"=w444) -> ()  [unwired: 2 in, 2 out]
            n117 = property on="QCM plot" class="WFChart (strict)"("History Data"=cluster{dbl, "Resistance out":dbl}[] []) -> ()  [unwired: 2 in, 2 out]
            n118 = property on="K-2100 (Ohm)" class="WFChart (strict)"("History Data"=w445) -> ()  [unwired: 2 in, 2 out]
            n119 = property on="arduino qcm 4" class="WFChart (strict)"("History Data"=w443) -> ()  [unwired: 2 in, 2 out]
            n120 = property on="K-2420" class="WFChart (strict)"("History Data"=w445) -> ()  [unwired: 2 in, 2 out]
            n121 = property on="pressure chart" class="WFChart (strict)"("History Data"=w444) -> ()  [unwired: 2 in, 2 out]
            n122 = property on="arduino qcm 2" class="WFChart (strict)"("History Data"=w443) -> ()  [unwired: 2 in, 2 out]
            n123 = property on="arduino qcm 5" class="WFChart (strict)"("History Data"=w443) -> ()  [unwired: 2 in, 2 out]
          }
          event "Sequence cluster.Clear sequence": Value Change {
            n124 = event-data() -> ()  [unwired: 1 in, 1 out]
            n125 = property on="User-defined\nsequence" class="Tbl (strict)"("Value"=string[][] []) -> ()  [unwired: 2 in, 2 out]
          }
          event "Sequence cluster.Save sequence": Value Change {
            n126 = event-data() -> ()  [unwired: 1 in, 1 out]
            n127 = call-poly <vilib>:"Write To Spreadsheet File.vi"("2D data"=w447) -> ()  [unwired: 7 in, 1 out]
          }
          event "Sequence cluster.Import sequence file": Value Change {
            n128 = event-data() -> ()  [unwired: 1 in, 1 out]
            n129 = call-poly <vilib>:"Read From Spreadsheet File.vi"() -> ("all rows"=w448:string[][])  [unwired: 7 in, 4 out]
            n130 = property on="User-defined\nsequence" class="Tbl (strict)"("Value"=w448) -> ()  [unwired: 2 in, 2 out]
          }
        }
        n131 = Unbundle(w291) -> ("press/RH/gas/vapor"=w290:T33, "Cluster"=w289:T34)
        n132 = Divide(x=w384, y=T11 {"f"=1000000.0, "f"=1000000.0, "f"=1000000.0, "f"=1000000.0, "f"=1000000.0}) -> (x/y=w359:T11)
        n133 = Unbundle(w289) -> ("Valve position (%)"=w287:dbl, "read pressure"=w281:dbl, "read vapor flow"=w286:dbl, "read gas flow"=w285:dbl)
        n134 = case shown="True" w348 {
          tunnel: w359 -> [_ w427]
          frame False {
          }
          frame True {
            n135 = Unbundle(w427) -> ("f"=w426:dbl, "f"=w425:dbl, "f"=w424:dbl, "f"=w423:dbl, "f"=w422:dbl)
            n136 = Bundle("f"=w426, "f"=w426, "f"=w425, "f"=w425, "f"=w424, "f"=w424, "f"=w423, "f"=w423, "f"=w422, "f"=w422) -> (→"ArduinoQCM\ncluster":T35)  [unwired: 1 in]
          }
        }
        n137 = Unbundle("Data logging settings") -> ("Save during sequence only"=w370:bool, "Save now"=w372:bool, "sec between data points"=w358:dbl, "Save sample names"=w309:T36, "Experiment Notes"=w308:string)  [unwired: 1 out]
        n138 = property on="Valve position (%)" class="DigNum (strict)"("Value"=w287) -> ()  [unwired: 2 in, 2 out]
        n139 = Subtract(x=w356, y=w334) -> (x-y=w355:dbl)
        n140 = property on="read pressure" class="DigNum (strict)"("Value"=w281) -> ()  [unwired: 2 in, 2 out]
        n141 = And(x=w288, y=w370) -> (x .and. y?=w369:bool)
        n142 = Bundle("read pressure"=w281) -> (w280:cluster{"read pressure":dbl})  [unwired: 1 in]
        n143 = Divide(x=w355, y=60.0) -> (x/y=w326:dbl)
        "Elapsed time (min)" <- w326
        n144 = call "data_headers_subVI.vi"("Experiment Notes"=w308, "Sample names"=w309) -> ("data headers"=w385:string[])  [unwired: 9 in]
        n145 = property on="read vapor flow" class="DigNum (strict)"("Value"=w286) -> ()  [unwired: 2 in, 2 out]
        n146 = Multiply(x=w358, y=u32 1000 ("x")) -> (x*y=w397:dbl)
        n147 = Or(x=w369, y=w372) -> (x .or. y?=w366:bool)
        "saving data?" <- w366
        n148 = Wait (ms)(milliseconds to wait=w397) -> ()  [unwired: 1 out]
        n149 = property on="read gas flow" class="DigNum (strict)"("Value"=w285) -> ()  [unwired: 2 in, 2 out]
        n150 = property on="pressure chart" class="WFChart (strict)"("Value"=w280) -> ()  [unwired: 2 in, 2 out]
        n151 = Get Date/Time In Seconds() -> (seconds since 1Jan1904=w419:timestamp)
        n152 = Number To Engineering String ("elapsed time (min)")(4:w326) -> (0:w331:string)  [unwired: 3 in]
        n153 = Unbundle(w303) -> ("current  step # in"=w277:i32, "sequence end time in"=w302:timestamp, "Boolean"=w301:bool)
        n154 = Format Date/Time String(time format string (%c)="%Y-%m-%d %H:%M:%S%2u", seconds (now)=w419) -> (date/time string=w394:string)  [unwired: 1 in]
        n155 = Unbundle(w339) -> ("String data out"=w330:string, w329:string, w328:string, w327:string)
        n156 = Unbundle(w390) -> ("String"=w332:string, "String"=w396:string, "String"=w395:string)
        n157 = Unbundle(w323) -> ("String"=w322:string, "String"=w321:string)
        n158 = Unbundle(w290) -> ("pressure"=w382:string, "RH"=w381:string, "gas flow"=w380:string, "vapor flow"=w379:string)
        n159 = Unbundle ("arduino 1-6")(w391) -> ("f"=w275:string, "f"=w389:string, "f"=w388:string, "f"=w387:string, "f"=w386:string)
        n160 = Increment(x=w277) -> (x+1=w276:i32)
        n161 = Build Array(w394, w331, w330, w329, w328, w327, w332, w396, w395, w322, w321, w382, w381, w380, w379, w274, w275, w389, w388, w387, w386) -> (w402:string[])
        n162 = property on="Current\nstep" class="DigNum (strict)"("Value"=w276) -> ()  [unwired: 2 in, 2 out]
        "State date/time" <- w325
      }
      n163 = Unbundle(w84) -> (w83:bool, "VISA resource name out"=w82:refnum<visa-resource-name>, "error out"=w81:errorcluster)
      n164 = Unbundle(w80) -> ("Boolean"=w79:bool, "VISA out"=w78:refnum<visa-resource-name>, "error out"=w77:errorcluster)
      n165 = call-poly <vilib>:"Write To Spreadsheet File.vi"("1D data"=w48, "file path (dialog if empty)"=w65) -> ("new file path (Not A Path if cancelled)"=w69:path)  [unwired: 6 in]
      n166 = Unbundle(w58) -> (w63:bool, "VISA resource name out"=w62:refnum<visa-resource-name>, "error out"=w61:errorcluster)
      n167 = Unbundle(w25) -> ("Boolean"=w24:bool, "DAQ IDs in"=w23:T37)
      n168 = call "arduino_close_subIV.vi"("arduino 1-6 addresses and errors out"=w50, "arduinos on?"=w49) -> ()  [unwired: 10 in]
      n169 = case shown="True" w41 {
        tunnel: w40 -> [_ w97]
        tunnel: w39 -> [w94 w96]
        tunnel: [w94 w95] -> w38
        frame False {
        }
        frame True {
          n170 = call "Close.vi"("VISA resource name"=w97, "error in (no error)"=w96) -> ("error out"=w95:errorcluster)  [unwired: 17 in]
        }
      }
      n171 = Unbundle(w75) -> ("Boolean"=w74:bool, "VISA resource name out"=w73:refnum<visa-resource-name>, "error out"=w72:errorcluster)
      n172 = case shown="True" w24 {
        tunnel: w23 -> [_ w126]
        tunnel: [errorcluster {"status"=FALSE, "code"=0, "source"=""} ("error out") w113] -> w33
        frame False {
        }
        frame True {
          n173 = Unbundle(w126) -> ("task out"=w125:refnum<k21>, "error out"=w124:errorcluster, "task out"=w123:refnum<k21>, "error out"=w122:errorcluster, "task out"=w121:refnum<k21>, "error out"=w120:errorcluster, "VISA Refnum out"=w119:refnum<visa-resource-name>, "error out"=w118:errorcluster)
          n174 = disable-structure shown="Disabled" {
            disable-tunnel: [w135 _] -> w117
            disable-tunnel: w125 -> [w134 _]
            disable-tunnel: w124 -> [w133 _]
            frame Disabled {
              n175 = call <vilib>:"DAQmx Stop Task.vi"("task/channels in"=w134, "error in"=w133) -> ("task out"=w136:refnum<k21>, "error out"=w137:errorcluster)  [unwired: 12 in]
              n176 = call <vilib>:"DAQmx Clear Task.vi"("task in"=w136, "error in"=w137) -> ("error out"=w135:errorcluster)  [unwired: 13 in]
            }
            frame Enabled {
            }
          }
          n177 = call <vilib>:"DAQmx Stop Task.vi"("task/channels in"=w123, "error in"=w122) -> ("task out"=w130:refnum<k21>, "error out"=w129:errorcluster)  [unwired: 12 in]
          n178 = call <vilib>:"DAQmx Stop Task.vi"("task/channels in"=w121, "error in"=w120) -> ("task out"=w131:refnum<k21>, "error out"=w132:errorcluster)  [unwired: 12 in]
          n179 = VISA Clear(VISA resource name=w119, error in (no error)=w118) -> (VISA resource name out=w128:refnum<visa-resource-name>, error out=w127:errorcluster)
          n180 = VISA Close(VISA resource name=w128, error in (no error)=w127) -> (error out=w114:errorcluster)
          n181 = call <vilib>:"DAQmx Clear Task.vi"("task in"=w130, "error in"=w129) -> ("error out"=w116:errorcluster)  [unwired: 13 in]
          n182 = call <vilib>:"DAQmx Clear Task.vi"("task in"=w131, "error in"=w132) -> ("error out"=w115:errorcluster)  [unwired: 13 in]
          n183 = Merge Errors(w117, w116, w115, w114) -> (w113:errorcluster)
        }
      }
      n184 = case shown="True" w83 {
        tunnel: w82 -> [_ w248]
        tunnel: w81 -> [w245 w247]
        tunnel: [w245 w246] -> w85
        frame False {
        }
        frame True {
          n185 = call "Enable Output.vi"("error in (no error)"=w247, "Enable Output (T: Enable)"=FALSE, "VISA resource name"=w248) -> ("error out"=w249:errorcluster, "VISA resource name out"=w251:refnum<visa-resource-name>)  [unwired: 7 in]
          n186 = call "Close.vi"("error in (no error)"=w249, "VISA resource name"=w251) -> ("error out"=w246:errorcluster)  [unwired: 9 in]
        }
      }
      n187 = case shown="True" w63 {
        tunnel: w62 -> [_ w161]
        tunnel: w61 -> [w159 w160]
        tunnel: [w159 w162] -> w57
        frame False {
        }
        frame True {
          n188 = call "Enable Output.vi"("error in (no error)"=w160, "Enable Output (F:Off)"=FALSE ("Output (F:Off)"), "VISA resource name"=w161) -> ("error out"=w163:errorcluster, "VISA resource name out"=w164:refnum<visa-resource-name>)  [unwired: 7 out]
          n189 = call "Close.vi"("error in (no error)"=w163, "VISA resource name"=w164) -> ("error out"=w162:errorcluster)  [unwired: 9 out]
        }
      }
      n190 = case shown="True" w79 {
        tunnel: w77 -> [w231 w234]
        tunnel: [w231 w233] -> w86
        tunnel: w78 -> [_ w232]
        frame False {
        }
        frame True {
          n191 = call "srsQcm200Close.vi"("error in"=w234, "Visa in"=w232) -> ("error out"=w233:errorcluster)  [unwired: 3 in]
        }
      }
      n192 = call-poly <vilib>:"Write To Spreadsheet File.vi"("append to file? (new file:F)"=TRUE, "2D data"=w52, "file path (dialog if empty)"=w69) -> ()  [unwired: 5 in, 1 out]
      n193 = case shown="True" w74 {
        tunnel: w73 -> [_ w201]
        tunnel: w72 -> [w198 w200]
        tunnel: [w198 w199] -> w71
        frame False {
        }
        frame True {
          n194 = VISA Close(VISA resource name=w201, error in (no error)=w200) -> (error out=w199:errorcluster)
        }
      }
      n195 = Merge Errors(w57, w71, w85, w38, w86, w32) -> (w92:errorcluster)
      n196 = call <vilib>:"Simple Error Handler.vi"("error in (no error)"=w33) -> ()  [unwired: 4 in, 5 out]
      n197 = call <vilib>:"Simple Error Handler.vi"("error in (no error)"=w92) -> ()  [unwired: 4 in, 5 out]
    }
  }
